vi "woo.vi"() -> ()   [LabVIEW 2009]
doc: "This example demonstrates some fundamental concepts for the 3D picture control. Concepts covered include:\n\n-Object creation\n-Texturing\n-Object movement\n-Object hierarchy"
uses:
  <vilib>/Utility/miscctls.llb/LVRectTypeDef.ctl
  <vilib>/Utility/inputDevices.llb/mouseAcquire.vi
  <vilib>/picture/3D Picture Control/NI_3D Picture Control.lvlib
  User32.dll
panel:
  in  "Paddle Size":sgl=20.0
  out "Cluster 2":cluster{"x":dbl, "x":dbl, "x":dbl}
  out "Cluster":cluster{"x":dbl, "x":dbl, "x":dbl}
  in  "brick size":sgl=2.0
  in  "brick number y":i32=5
  in  "Brick number x":i32=5
  in  "Render Dest":enum16{"Scene Window", "Scene Display"}(ring)
  in  "Camera Controller":enum16{"None", "Spherical", "Flying"}(ring)=enum."Spherical"
  out "Scene Display":refnum<vi>(3d-picture)
  in  "stop":bool
  # "Select 'Render Dest'\nbefore running!"
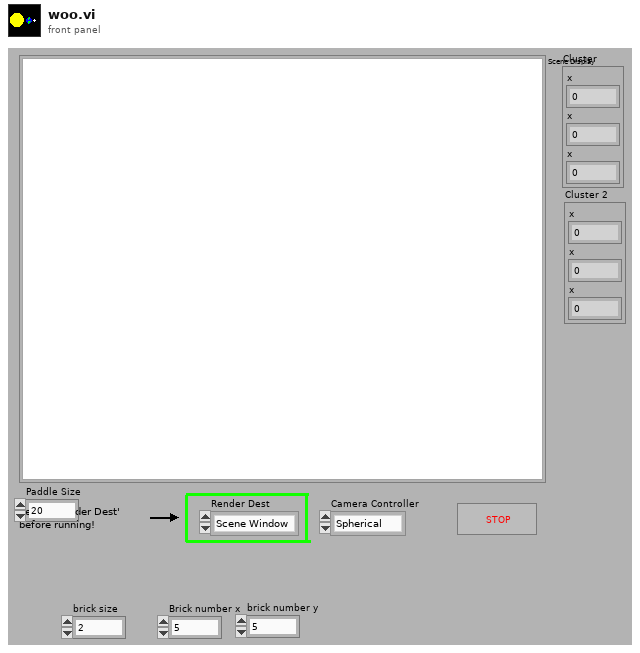
[diagram p1: front panel]
types:
  T1 = cluster{"Red":sgl, "Green":sgl, "Blue":sgl, "Alpha":sgl}
  T2 = enum16{"Normal Bin", "Opaque Bin", "Transparent Bin"}
  T3 = typedef "LVRectTypeDef.ctl" = cluster{"Left":i16, "Top":i16, "Right":i16, "Bottom":i16}
  T4 = enum16{"Open", "Minimized", "Maximized", "Hidden"}
  T5 = enum16{"As a Decal", "With Modulation", "With Blending", "As a replacement"}
  T6 = typedef "imagedata.ctl" = cluster{"image type":i32, "image depth":i32, "image":u8[], "mask":u8[], "colors":u32[], "Rectangle":cluster{"left":i16, "top":i16, "right":i16, "bottom":i16}}
  T7 = enum16{"No Filtration", "Linear Filtration", "Simple Mipmap Filtration", "Bilinear Filtration", "Trilinear Filtration"}
  T8 = cluster{"Horizontal":i32, "Vertical":i32, "Scrolling":i32}
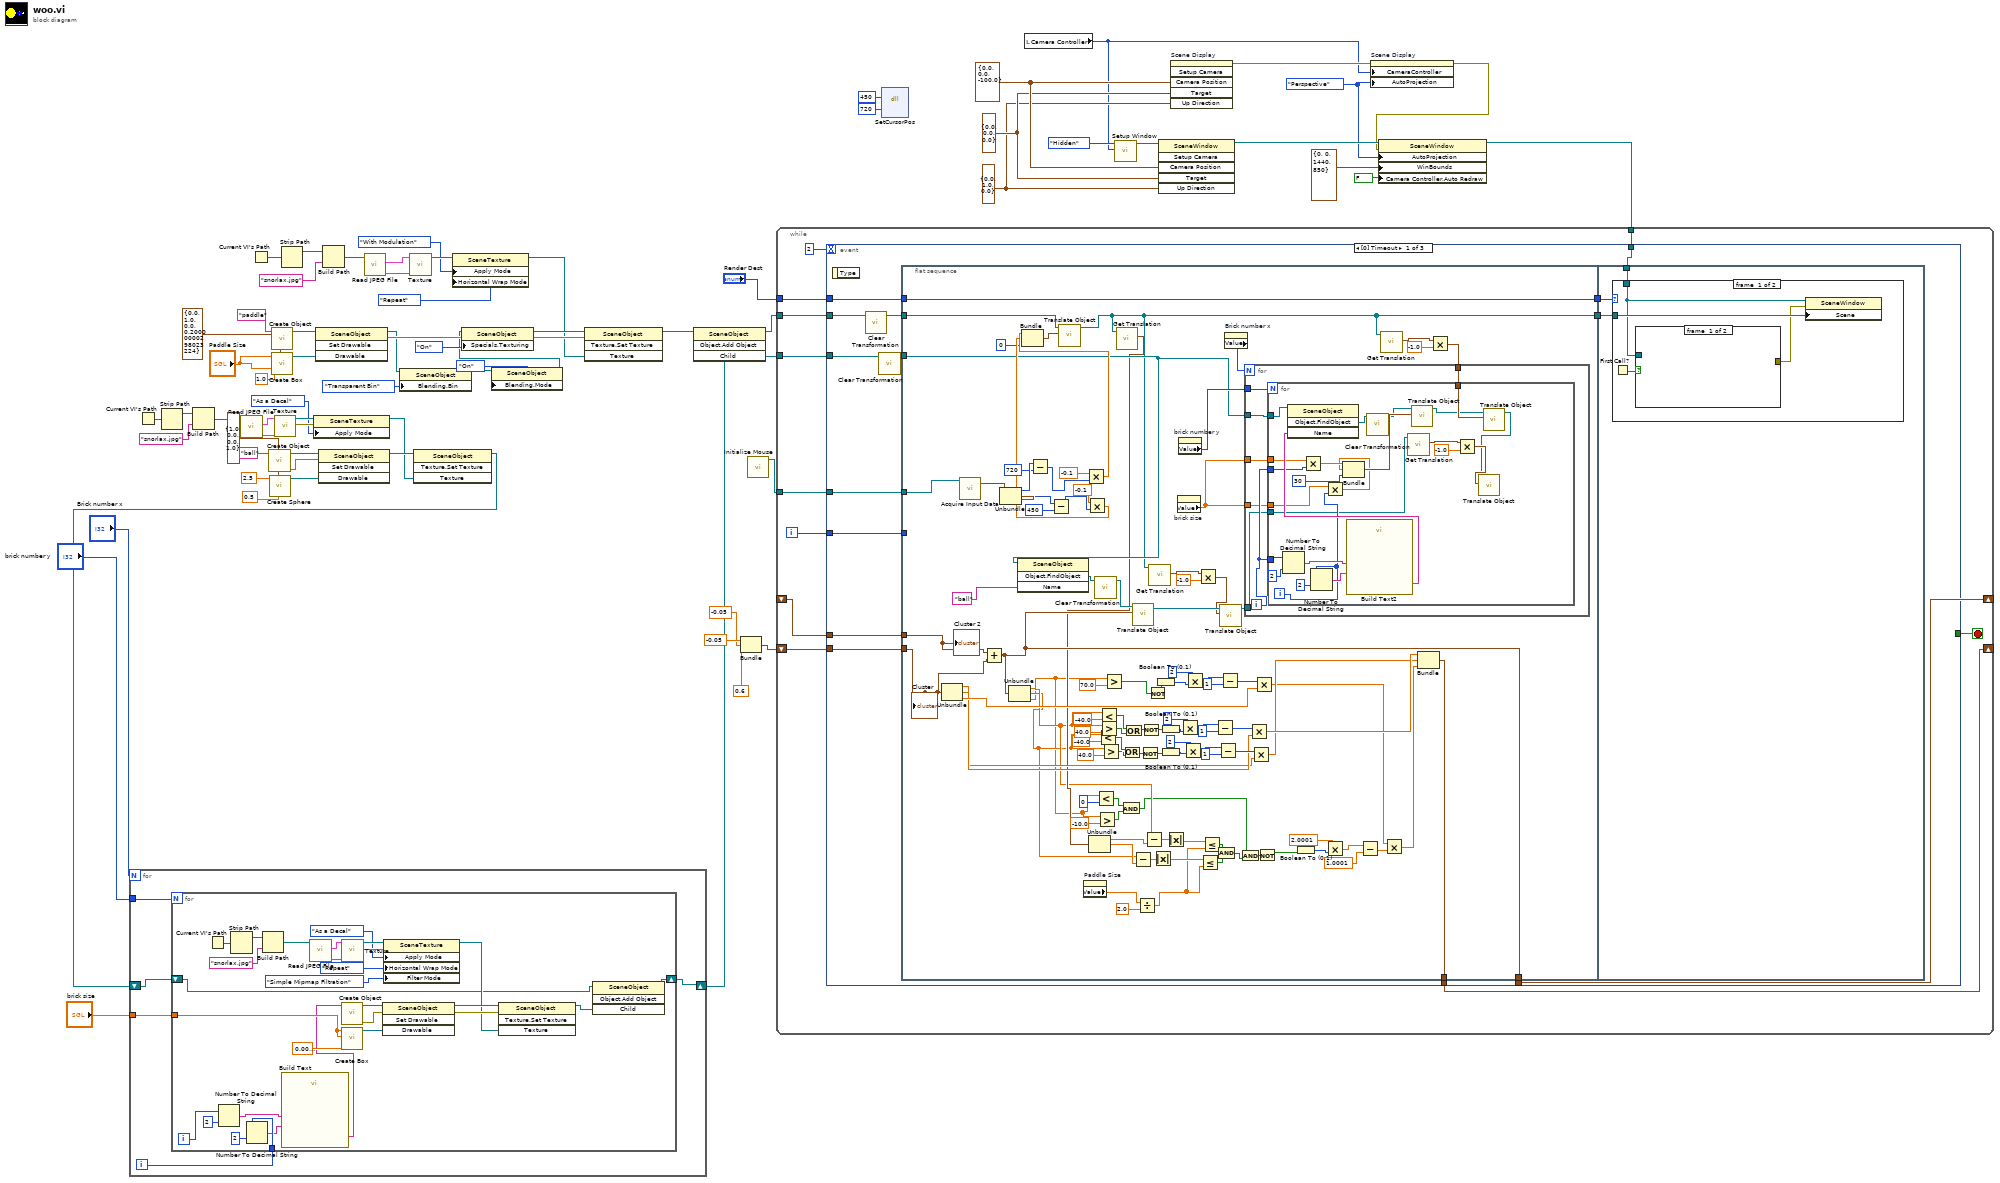
[diagram p0: block diagram]
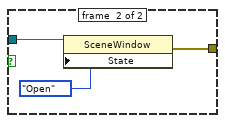
[diagram p2: hidden frame]
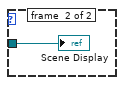
[diagram p3: hidden frame]
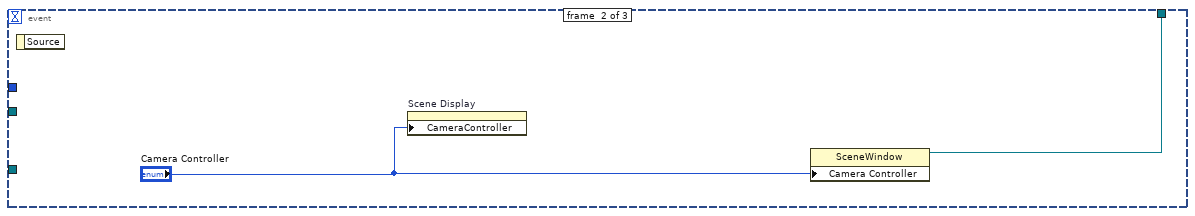
[diagram p4: hidden frame]
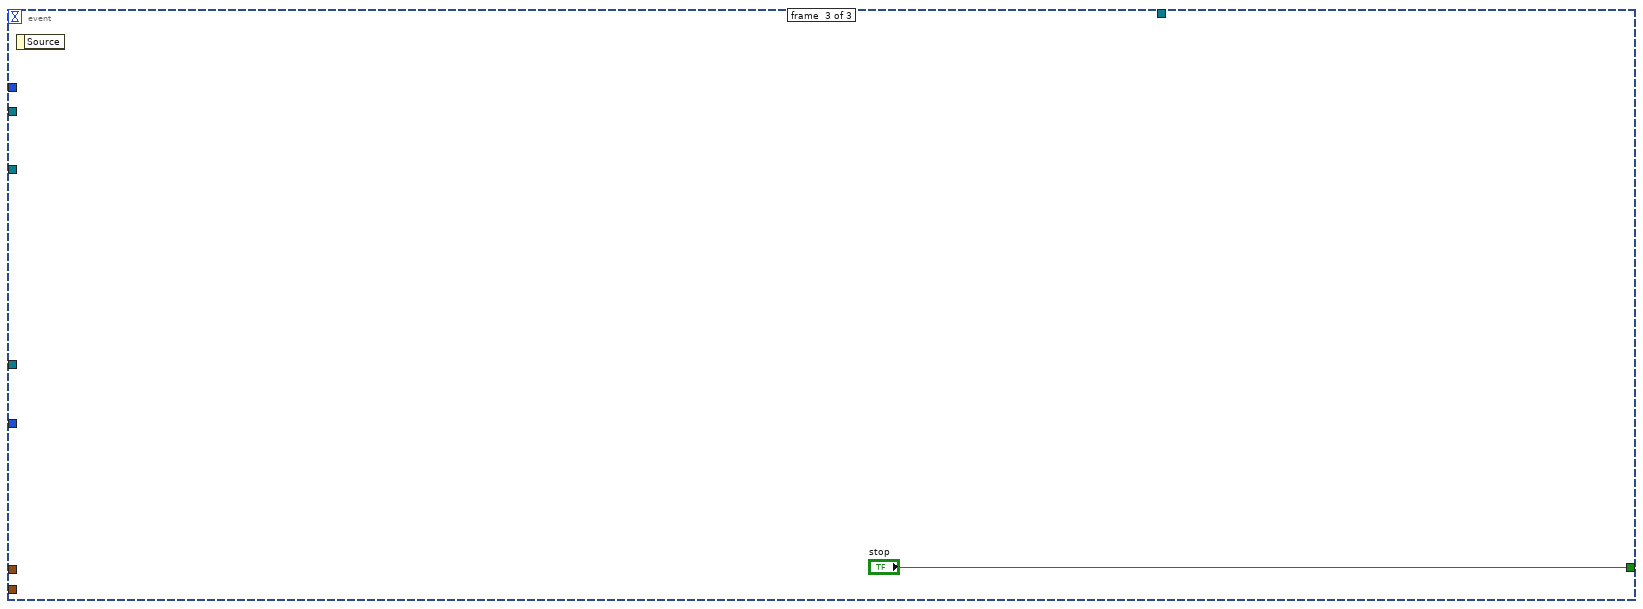
[diagram p5: hidden frame]
diagram:
  w28 = enum16{"None", "Perspective", "Orthographic"}."Perspective" ("Auto Projection Mode")
  w31 = cluster{"X":sgl, "Y":sgl, "Z":sgl} {"X"=0.0, "Y"=1.0, "Z"=0.0} ("Up Direction")
  w32 = cluster{"X":sgl, "Y":sgl, "Z":sgl} {"X"=0.0, "Y"=0.0, "Z"=0.0} ("Target")
  w33 = cluster{"X":sgl, "Y":sgl, "Z":sgl} {"X"=0.0, "Y"=0.0, "Z"=-100.0} ("Camera Position")
  n1 = Current VI's Path() -> (path=w37:path)
  n2 = Strip Path(path=w37) -> (stripped path=w38:path)  [unwired: 1 out]
  n3 = Build Path(base path=w38, name or relative path="snorlax.jpg" ("Name")) -> (appended path=w36:path)
  n4 = call <vilib>:"Read JPEG File.vi"("path to JPEG file"=w36) -> ("error out"=w66:errorcluster, "image data"=w65:T6)  [unwired: 1 in, 8 out]
  n5 = Current VI's Path() -> (path=w43:path)
  n6 = call <vilib>:"Create Object.vi"("Name"="ball") -> ("error out"=w45:errorcluster, "Scene:New Object"=w47:refnum<vi>)  [unwired: 1 in, 8 out]
  n7 = call <vilib>:"Create Sphere.vi"("Detail"=sgl 0.5, "Color"=T1 {"Red"=1.0, "Green"=0.0, "Blue"=0.0, "Alpha"=1.0}, "Radius"=sgl 2.5) -> ("New Sphere Refnum"=w46:refnum<vi>)  [unwired: 7 in, 1 out]
  n8 = call <vilib>:"Create Object.vi"("Name"="paddle") -> ("Scene:New Object"=w70:refnum<vi>)  [unwired: 1 in, 9 out]
  n9 = call <vilib>:"Create Box.vi"("Color"=T1 {"Red"=0.0, "Green"=1.0, "Blue"=0.0, "Alpha"=0.2}, "Length Z"=sgl 1.0 ("Detail"), "Length Y"="Paddle Size", "Length X"="Paddle Size") -> ("New Box Refnum"=w68:refnum<vi>)  [unwired: 6 in, 1 out]
  n10 = call <vilib>:"Texture.vi"("error in (no error)"=w66, "Image"=w65) -> ("error out"=w52:errorcluster, "New Texture Refnum"=w53:refnum<vi>)  [unwired: 8 out]
  n11 = Strip Path(path=w43) -> (stripped path=w42:path)  [unwired: 1 out]
  n12 = property class="SceneTexture"(reference=w53, error in=w52, "Apply Mode"=T5."As a Decal") -> (reference out=w35:refnum<vi>)  [unwired: 1 out]
  n13 = invoke class="SceneObject" method="Set Drawable"(reference=w70, "Drawable"=w68) -> (reference out=w19:refnum<vi>, error out=w59:errorcluster)  [unwired: 2 in, 2 out]
  n14 = invoke class="SceneObject" method="Set Drawable"(reference=w47, error in=w45, "Drawable"=w46) -> (reference out=w44:refnum<vi>)  [unwired: 1 in, 3 out]
  n15 = Build Path(base path=w42, name or relative path="snorlax.jpg" ("Name")) -> (appended path=w40:path)
  n16 = call <vilib>:"Read JPEG File.vi"("path to JPEG file"=w40) -> ("error out"=w64:errorcluster, "image data"=w67:T6)  [unwired: 1 in, 8 out]
  n17 = property class="SceneObject"(reference=w19, "Blending.Bin"=T2."Transparent Bin" ("Blending:Bin")) -> (reference out=w17:refnum<vi>)  [unwired: 1 in, 1 out]
  n18 = call <vilib>:"Texture.vi"("error in (no error)"=w64, "Image"=w67) -> ("New Texture Refnum"=w56:refnum<vi>)  [unwired: 9 out]
  n19 = invoke class="SceneObject" method="Texture.Set Texture"(reference=w44, "Texture"=w35) -> (reference out=w10:refnum<vi>)  [unwired: 2 in, 3 out]
  n20 = for {
    N: "Brick number x" -> [_]
    tunnel: "brick number y" -> [w77]
    tunnel: "brick size" -> [w76]
    shift-right: [w74] -> w11
    shift-left: w10 -> [w73]
    i -> [w75]
    n21 = for {
      N: w77 -> [_]
      tunnel: w76 -> [w88]
      tunnel: w75 -> [w83]
      shift-right: [w79] -> w74
      shift-left: w73 -> [w78]
      i -> [w85]
      n22 = Current VI's Path() -> (path=w94:path)
      n23 = Number To Decimal String(number=w85, width (-)=i16 2) -> (decimal integer string=w81:string)
      n24 = Strip Path(path=w94) -> (stripped path=w93:path)  [unwired: 1 out]
      n25 = Number To Decimal String(number=w83, width (-)=i16 2) -> (decimal integer string=w82:string)
      n26 = Build Path(base path=w93, name or relative path="snorlax.jpg" ("Name")) -> (appended path=w91:path)
      n27 = call "Build Text"("x"=w81, "y"=w82) -> ("Result"=w87:string)  [unwired: 12 in, 1 out]
      n28 = call <vilib>:"Read JPEG File.vi"("path to JPEG file"=w91) -> ("error out"=w103:errorcluster, "image data"=w102:T6)  [unwired: 1 in, 8 out]
      n29 = call <vilib>:"Create Object.vi"("Name"=w87) -> ("error out"=w105:errorcluster, "Scene:New Object"=w106:refnum<vi>)  [unwired: 1 in, 8 out]
      n30 = call <vilib>:"Create Box.vi"("Length Z"=sgl 0.01 ("Detail"), "Length Y"=w88, "Length X"=w88) -> ("New Box Refnum"=w104:refnum<vi>)  [unwired: 7 in, 1 out]
      n31 = call <vilib>:"Texture.vi"("error in (no error)"=w103, "Image"=w102) -> ("error out"=w98:errorcluster, "New Texture Refnum"=w99:refnum<vi>)  [unwired: 8 out]
      n32 = invoke class="SceneObject" method="Set Drawable"(reference=w106, error in=w105, "Drawable"=w104) -> (reference out=w101:refnum<vi>, error out=w100:errorcluster)  [unwired: 1 in, 2 out]
      n33 = property class="SceneTexture"(reference=w99, error in=w98, "Apply Mode"=T5."As a Decal", "Horizontal Wrap Mode"=enum16{"Clamp", "Repeat"}."Repeat", "Filter Mode"=T7."Simple Mipmap Filtration") -> (reference out=w96:refnum<vi>)  [unwired: 1 out]
      n34 = invoke class="SceneObject" method="Texture.Set Texture"(reference=w101, error in=w100, "Texture"=w96) -> (reference out=w80:refnum<vi>)  [unwired: 1 in, 3 out]
      n35 = invoke class="SceneObject" method="Object.Add Object"(reference=w78, "Child"=w80) -> (reference out=w79:refnum<vi>)  [unwired: 2 in, 3 out]
    }
  }
  n36 = property class="SceneTexture"(reference=w56, "Apply Mode"=T5."With Modulation", "Horizontal Wrap Mode"=enum16{"Clamp", "Repeat"}."Repeat") -> (reference out=w54:refnum<vi>)  [unwired: 1 in, 1 out]
  n37 = property class="SceneObject"(reference=w17, "Blending.Mode"=enum16{"Inherit Value", "Off", "On"}."On" ("Blending:Mode")) -> (reference out=w15:refnum<vi>)  [unwired: 1 in, 1 out]
  n38 = property class="SceneObject"(reference=w15, error in=w59, "Specials.Texturing"=enum16{"Inherit Value", "Off", "On"}."On" ("Specials:Texturing")) -> (reference out=w60:refnum<vi>, error out=w58:errorcluster)
  n39 = invoke class="SceneObject" method="Texture.Set Texture"(reference=w60, error in=w58, "Texture"=w54) -> (reference out=w63:refnum<vi>)  [unwired: 1 in, 3 out]
  n40 = invoke class="SceneObject" method="Object.Add Object"(reference=w63, "Child"=w11) -> (reference out=w62:refnum<vi>, "Child"=w61:refnum<vi>)  [unwired: 2 in, 2 out]
  n41 = Bundle("x"=-0.05, "x"=-0.05, "x"=0.6) -> (w4:cluster{"x":dbl, "x":dbl, "x":dbl})  [unwired: 1 in]
  n42 = call <vilib>:"Initialize Mouse.vi"() -> ("device ID"=w8:refnum<k1>)  [unwired: 10 in, 1 out]
  n43 = dll-call lib="User32.dll" fn="SetCursorPos"(720, 450) -> ()  [unwired: 5 in, 3 out]
  n44 = local read "Camera Controller"() -> (w24:enum16{"None", "Spherical", "Flying"})
  n45 = call <vilib>:"Setup Window.vi"("Camera Controller"=w24, "Window State"=T4."Hidden") -> ("New Window Refnum"=w26:refnum<vi>)  [unwired: 1 in, 8 out]
  n46 = invoke class="SceneWindow" method="Setup Camera"(reference=w26, "Camera Position"=w33, "Target"=w32, "Up Direction"=w31) -> (reference out=w72:refnum<vi>)  [unwired: 2 in, 5 out]
  n47 = invoke on="Scene Display" class="SceneGraphDisp (strict)" method="Setup Camera"("Camera Position"=w33, "Target"=w32, "Up Direction"=w31) -> (error out=w30:errorcluster)  [unwired: 3 in, 5 out]
  n48 = property on="Scene Display" class="SceneGraphDisp (strict)"(error in=w30, "CameraController"=w24, "AutoProjection"=w28) -> (error out=w29:errorcluster)  [unwired: 1 in, 1 out]
  n49 = property class="SceneWindow"(reference=w72, error in=w29, "AutoProjection"=w28, "WinBounds"=T3 {"Left"=0, "Top"=0, "Right"=1440, "Bottom"=850} ("Window Bounds"), "Camera Controller.Auto Redraw"=FALSE ("Camera Controller:Auto Redraw")) -> (reference out=w22:refnum<vi>)  [unwired: 1 out]
  n50 = while {
    tunnel: w22 -> [w118]
    tunnel: w62 -> [w117]
    tunnel: w61 -> [w116]
    tunnel: "Render Dest" -> [w113]
    tunnel: w8 -> [w111]
    shift-right: [w108] -> _
    shift-left: _ -> [w110]
    shift-right: [w107] -> _
    shift-left: w4 -> [w109]
    i -> [w112]
    stop <- w114 stop-if-true
    n51 = event shown="[0] Timeout" {
      selector: _ -> [_ _ _]
      dyn-events: _ -> [_ _ _]
      timeout: 2 -> [_ _ _]
      tunnel: w112 -> [w131 _ _]
      tunnel: w118 -> [w130 w277 _]
      tunnel: w117 -> [w125 _ _]
      tunnel: w116 -> [w129 _ _]
      tunnel: [_ _ "stop"] -> w114
      tunnel: w113 -> [w127 _ _]
      tunnel: w111 -> [w123 _ _]
      tunnel: w110 -> [w122 _ _]
      tunnel: w109 -> [w121 _ _]
      tunnel: [w120 _ _] -> w108
      tunnel: [w119 _ _] -> w107
      event #0 {
        n52 = event-data() -> ()  [unwired: 2 out]
        n53 = call <vilib>:"Clear Transformation.vi"("Object Refnum In"=w125) -> ("Object Refnum Out"=w124:refnum<vi>)  [unwired: 1 in, 9 out]
        n54 = call <vilib>:"Clear Transformation.vi"("Object Refnum In"=w129) -> ("Object Refnum Out"=w126:refnum<vi>)  [unwired: 1 in, 9 out]
        n55 = flat-sequence {
          tunnel: w131 -> [_]
          tunnel: [w164] -> w132
          tunnel: w124 -> [w221]
          tunnel: [w233] -> w128
          tunnel: w127 -> [w233]
          tunnel: w126 -> [w174]
          tunnel: w123 -> [w229]
          tunnel: w122 -> [w210]
          tunnel: w121 -> [w209]
          tunnel: [w208] -> w120
          tunnel: [w211] -> w119
          tunnel: w130 -> [w267]
          tunnel: w132 -> [w266]
          tunnel: w128 -> [w265]
          frame #0 {
            n56 = Unbundle(w209) -> ("x"=w188:dbl, "x"=w187:dbl, "x"=w201:dbl)
            n57 = call-poly <vilib>:"Acquire Input Data.vi"("device ID"=w229) -> ("axis info"=w228:T8)  [unwired: 15 in, 3 out]
            n58 = Add(x=w210, y=w209) -> (x+y=w208:cluster{"x":dbl, "x":dbl, "x":dbl})
            n59 = Unbundle(w228) -> ("Horizontal"=w220:i32, "Vertical"=w216:i32)  [unwired: 1 out]
            n60 = Unbundle(w208) -> ("x"=w159:dbl, "x"=w158:dbl, "x"=w137:dbl)
            n61 = invoke class="SceneObject" method="Object.FindObject"(reference=w174, "Name"="ball") -> ("FindObject"=w213:refnum<vi>)  [unwired: 2 in, 3 out]
            n62 = Subtract(x=w220, y=720) -> (x-y=w219:i32)
            n63 = Subtract(x=w216, y=450) -> (x-y=w215:i32)
            n64 = property on="Paddle Size" class="DigNum (strict)"() -> ("Value"=w134:sgl)  [unwired: 2 in, 2 out]
            n65 = Multiply(x=-0.1, y=w219) -> (x*y=w224:dbl)
            n66 = Multiply(x=-0.1, y=w215) -> (x*y=w223:dbl)
            n67 = Bundle(w224, w223, "width (-)"=i16 0) -> (w225:cluster{dbl, dbl, "width (-)":i16})  [unwired: 1 in]
            n68 = call <vilib>:"Translate Object.vi"("Translation"=w225, "Scene.Object In"=w221) -> ("Scene.Object Out"=w164:refnum<vi>)  [unwired: 1 in, 8 out]
            n69 = call <vilib>:"Clear Transformation.vi"("Object Refnum In"=w213) -> ("Object Refnum Out"=w212:refnum<vi>)  [unwired: 1 in, 9 out]
            n70 = Less?(x=w137, y=i8 0) -> (x < y?=w139:bool)
            n71 = Greater?(x=w137, y=-10.0) -> (0:w140:bool)
            n72 = Less?(x=w158, y=-40.0) -> (x < y?=w180:bool)
            n73 = Greater?(x=w159, y=40.0) -> (0:w182:bool)
            n74 = Less?(x=w159, y=-40.0) -> (x < y?=w183:bool)
            n75 = Greater?(x=w158, y=40.0) -> (0:w170:bool)
            n76 = Greater?(x=w137, y=70.0) -> (0:w150:bool)
            n77 = call <vilib>:"Get Translation.vi"("Scene Object"=w164) -> ("Transformation:Get Translation"=w162:cluster{"X":sgl, "Y":sgl, "Z":sgl})  [unwired: 8 in, 2 out]
            n78 = Unbundle(w162) -> ("X"=w161:sgl, "Y"=w160:sgl)  [unwired: 1 out]
            n79 = And(x=w139, y=w140) -> (x .and. y?=w138:bool)
            n80 = Or(x=w180, y=w170) -> (x .or. y?=w166:bool)
            n81 = Or(x=w183, y=w182) -> (x .or. y?=w167:bool)
            n82 = call <vilib>:"Translate Object.vi"("Translation"=w208, "Scene.Object In"=w212) -> ("Scene.Object Out"=w173:refnum<vi>)  [unwired: 1 in, 8 out]
            n83 = Subtract(x=w158, y=w160) -> (x-y=w156:dbl)
            n84 = Divide(x=w134, y=2.0) -> (x/y=w133:dbl)
            n85 = Not(x=w166) -> (.not. x?=w165:bool)
            n86 = Not(x=w167) -> (.not. x?=w168:bool)
            n87 = Subtract(x=w159, y=w161) -> (x-y=w157:dbl)
            n88 = Not(x=w150) -> (.not. x?=w169:bool)
            n89 = call <vilib>:"Get Translation.vi"("Scene Object"=w164) -> ("Transformation:Get Translation"=w175:cluster{"X":sgl, "Y":sgl, "Z":sgl})  [unwired: 8 in, 2 out]
            n90 = Absolute Value(x=w156) -> (abs(x)=w154:dbl)
            n91 = Boolean To (0,1)(Boolean=w169) -> (0, 1=w206:i16)
            n92 = Boolean To (0,1)(Boolean=w168) -> (0, 1=w199:i16)
            n93 = Boolean To (0,1)(Boolean=w165) -> (0, 1=w193:i16)
            n94 = Absolute Value(x=w157) -> (abs(x)=w155:dbl)
            n95 = property on="brick size" class="DigNum (strict)"() -> ("Value"=w230:sgl)  [unwired: 2 in, 2 out]
            n96 = property on="brick number y" class="DigNum (strict)"() -> ("Value"=w232:i32)  [unwired: 2 in, 2 out]
            n97 = Multiply(x=i16 2, y=w199) -> (x*y=w197:i16)
            n98 = Multiply(x=i16 2, y=w193) -> (x*y=w191:i16)
            n99 = Multiply(x=i16 2, y=w206) -> (x*y=w204:i16)
            n100 = Multiply(x=w175, y=-1.0) -> (x*y=w172:cluster{"X":dbl, "Y":dbl, "Z":dbl})
            n101 = Less Or Equal?(x=w154, y=w133) -> (x <= y?=w152:bool)
            n102 = Less Or Equal?(x=w155, y=w133) -> (x <= y?=w153:bool)
            n103 = Subtract(x=w197, y=i16 1) -> (x-y=w195:i16)
            n104 = And(x=w153, y=w152) -> (x .and. y?=w151:bool)
            n105 = Subtract(x=w191, y=i16 1) -> (x-y=w189:i16)
            n106 = call <vilib>:"Translate Object.vi"("Translation"=w172, "Scene.Object In"=w173) -> ("Scene.Object Out"=w171:refnum<vi>)  [unwired: 1 in, 8 out]
            n107 = Subtract(x=w204, y=i16 1) -> (x-y=w202:i16)
            n108 = property on="Brick number x" class="DigNum (strict)"() -> ("Value"=w231:i32)  [unwired: 2 in, 2 out]
            n109 = And(x=w138, y=w151) -> (x .and. y?=w144:bool)
            n110 = Multiply(x=w195, y=w188) -> (x*y=w186:dbl)
            n111 = Multiply(x=w189, y=w187) -> (x*y=w185:dbl)
            n112 = Multiply(x=w202, y=w201) -> (x*y=w142:dbl)
            n113 = Not(x=w144) -> (.not. x?=w145:bool)
            n114 = Boolean To (0,1)(Boolean=w145) -> (0, 1=w149:i16)
            n115 = Multiply(x=2.0001, y=w149) -> (x*y=w147:dbl)
            n116 = Subtract(x=w147, y=1.0001) -> (x-y=w143:dbl)
            n117 = call <vilib>:"Get Translation.vi"("Scene Object"=w164) -> ("Transformation:Get Translation"=w178:cluster{"X":sgl, "Y":sgl, "Z":sgl})  [unwired: 8 in, 2 out]
            n118 = Multiply(x=w142, y=w143) -> (x*y=w141:dbl)
            n119 = Bundle(w186, w185, w141) -> (w211:cluster{dbl, dbl, dbl})  [unwired: 1 in]
            n120 = Multiply(x=w178, y=-1.0) -> (x*y=w177:cluster{"X":dbl, "Y":dbl, "Z":dbl})
            n121 = for {
              N: w231 -> [_]
              tunnel: w174 -> [w240]
              tunnel: w232 -> [w239]
              tunnel: w230 -> [w237]
              tunnel: w230 -> [w236]
              tunnel: w177 -> [w235]
              tunnel: w171 -> [w234]
              i -> [w238]
              n122 = for {
                N: w239 -> [_]
                tunnel: w240 -> [w264]
                tunnel: w238 -> [w259]
                tunnel: w238 -> [w253]
                tunnel: w237 -> [w252]
                tunnel: w236 -> [w249]
                tunnel: w235 -> [w247]
                tunnel: w234 -> [w243]
                i -> [w250]
                n123 = Number To Decimal String(number=w259, width (-)=i16 2) -> (decimal integer string=w260:string)
                n124 = Multiply(x=w252, y=w253) -> (x*y=w251:sgl)
                n125 = Number To Decimal String(number=w250, width (-)=i16 2) -> (decimal integer string=w261:string)
                n126 = Multiply(x=w249, y=w250) -> (x*y=w248:sgl)
                n127 = Bundle(w251, w248, "element"=30) -> (w256:cluster{sgl, sgl, "element":i32})  [unwired: 1 in]
                n128 = call "Build Text2"("x"=w260, "y"=w261) -> ("Result"=w258:string)  [unwired: 12 in, 1 out]
                n129 = invoke class="SceneObject" method="Object.FindObject"(reference=w264, "Name"=w258) -> ("FindObject"=w255:refnum<vi>)  [unwired: 2 in, 3 out]
                n130 = call <vilib>:"Clear Transformation.vi"("Object Refnum In"=w255) -> ("Object Refnum Out"=w254:refnum<vi>)  [unwired: 1 in, 9 out]
                n131 = call <vilib>:"Get Translation.vi"("Scene Object"=w243) -> ("Transformation:Get Translation"=w244:cluster{"X":sgl, "Y":sgl, "Z":sgl})  [unwired: 8 in, 2 out]
                n132 = call <vilib>:"Translate Object.vi"("Translation"=w256, "Scene.Object In"=w254) -> ("Scene.Object Out"=w242:refnum<vi>)  [unwired: 1 in, 8 out]
                n133 = Multiply(x=w244, y=-1.0) -> (x*y=w245:cluster{"X":dbl, "Y":dbl, "Z":dbl})
                n134 = call <vilib>:"Translate Object.vi"("Translation"=w247, "Scene.Object In"=w242) -> ("Scene.Object Out"=w241:refnum<vi>)  [unwired: 1 in, 8 out]
                n135 = call <vilib>:"Translate Object.vi"("Translation"=w245, "Scene.Object In"=w241) -> ()  [unwired: 1 in, 9 out]
              }
            }
            "Cluster" <- w209
            "Cluster 2" <- w210
          }
          frame #1 {
            n136 = case shown="\"Scene Display\"" w265 {
              tunnel: w267 -> [w270 _]
              tunnel: w266 -> [w271 w275]
              frame #0 {
                n137 = First Call?() -> (First Call?: T/F=w268:bool)
                n138 = case shown="True" w268 {
                  tunnel: w270 -> [_ w274]
                  tunnel: [_ w273] -> w269
                  frame #0 {
                  }
                  frame #1 {
                    n139 = property class="SceneWindow"(reference=w274, "State"=T4."Open" ("Window State")) -> (error out=w273:errorcluster)  [unwired: 1 in, 1 out]
                  }
                }
                n140 = property class="SceneWindow"(reference=w270, error in=w269, "Scene"=w271) -> ()  [unwired: 2 out]
              }
              frame #1 {
                "Scene Display" <- w275
              }
            }
          }
        }
      }
      event #1 {
        n141 = event-data() -> ()  [unwired: 2 out]
        n142 = property on="Scene Display" class="SceneGraphDisp (strict)"("CameraController"="Camera Controller") -> ()  [unwired: 2 in, 2 out]
        n143 = property class="SceneWindow"(reference=w277, "Camera Controller"="Camera Controller") -> ()  [unwired: 1 in, 2 out]
      }
      event #2 {
        n144 = event-data() -> ()  [unwired: 2 out]
      }
    }
  }
